vi "Config.vi"(8 "error in (no error)":errorcluster, 10 "Setting":T1={"Resolution (Digits)"=5.5, "Current Source (Amps)"=0.001, "Range"=2.0, "Measurement Type"=enum."DC Volts"} {"Range" format="%.2p"; "Current Source (Amps)" items=["1uA"=1e-06, "10uA"=1e-05, "100uA"=0.0001, "1mA"=0.001]; "Resolution (Digits)" items=["3 1/2"=3.5, "4 1/2"=4.5, "5 1/2"=5.5, "6 1/2"=6.5, "7 1/2"=7.5]}, 11 "DMM in":refnum<class "NI DMM4072.lvclass">) -> (0 "error out":errorcluster, 3 "DMM out":refnum<class "NI DMM4072.lvclass">)   [LabVIEW 2019, in "Concrete.lvlib" / "NI DMM4072.lvclass"]
uses:
  NI DMM4072.lvclass
  NI DMM4072.lvclass/NI DMM4072.ctl
  <instrlib>/niDMM/nidmm.llb/niDMM Configure Measurement Digits.vi
  Harware Abstraction/MultiIO/MIO.lvclass
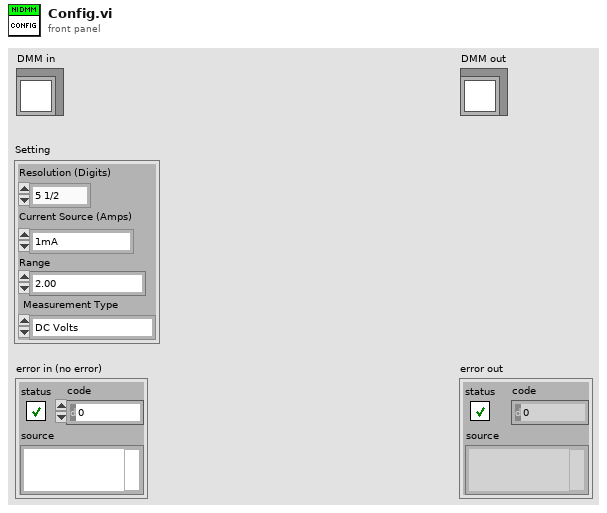
[diagram p1: front panel]
types:
  T1 = cluster{"Resolution (Digits)":dbl, "Current Source (Amps)":dbl, "Range":dbl, "Measurement Type":enum16{"DC Volts", "AC Volts", "DC Current", "AC Current", "2-wire Resistance", "4-wire Resistance", "Diode", "Frequency", "Period", "AC Volts DC Coupled", "Capacitance", "Inductance", "Temperature"}}
  T2 = enum16{"DC Volts", "AC Volts", "DC Current", "AC Current", "2-wire Resistance", "4-wire Resistance", "Diode", "Frequency", "Period", "AC Volts DC Coupled", "Capacitance", "Inductance", "Temperature"}
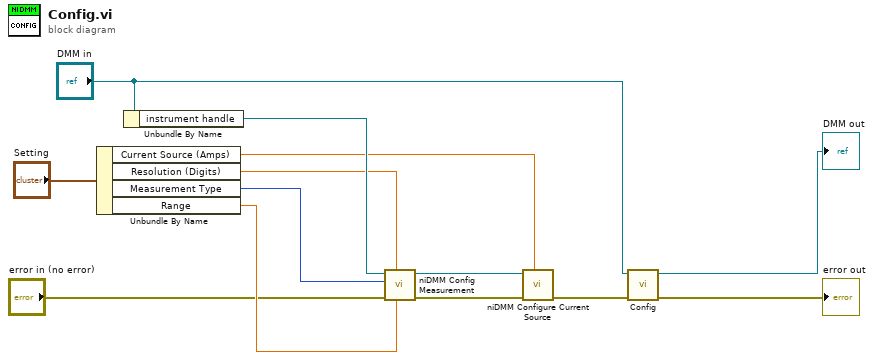
[diagram p0: block diagram]
diagram:
  n1 = Unbundle By Name("Setting") -> ("Current Source (Amps)"=w1:dbl, "Resolution (Digits)"=w8:dbl, "Measurement Type"=w6:T2, "Range"=w7:dbl)
  n2 = Unbundle By Name("DMM in") -> ("instrument handle"=w9:refnum<k15>)
  n3 = call-poly <instrlib>:"niDMM Config Measurement.vi"("Range"=w7, "Resolution in Digits"=w8, "error in (no error)"="error in (no error)", "Function"=w6, "instrument handle"=w9) -> ("error out"=w4:errorcluster, "instrument handle out"=w3:refnum<k15>)  [unwired: 5 in]
  n4 = call <instrlib>:"niDMM Configure Current Source.vi"("Current Source"=w1, "error in (no error)"=w4, "instrument handle"=w3) -> ("error out"=w2:errorcluster)  [unwired: 7 in, 1 out]
  n5 = call-parent "Config.vi"("error in (no error)"=w2, "DMM in"="DMM in") -> ("error out"=→"error out":errorcluster, "DMM out"=→"DMM out":refnum<class "NI DMM4072.lvclass">)  [unwired: 8 in]
